vi "Bar Code Reader_v5.vi"() -> ()   [LabVIEW 2016]
uses:
  <vilib>/NXT/Block Support/NXT_OutputPort.ctl
  <vilib>/NXT/Block Support/NXT_InputPort.ctl
  <vilib>/NXT/Dual Mode Library/Sensors/EV3_Color_Color.vi
  <vilib>/NXT/NXTIO Xnodes/NXTIONodeSubVIs/NXTMoveMotors.vi
  <vilib>/NXT/NXTIO Xnodes/NXTIONodeSubVIs/NXTMotorRunDistance.vi
  <vilib>/NXT/Dual Mode Library/Waits/Wait_Num.vi
  <vilib>/NXT/Subs/LVHSConnector.ctl
  <vilib>/NXT/NXTIO Xnodes/AddressXNode/NXTIOAddress.xnode
  <vilib>/NXT/NXTIO Xnodes/NXTIOXNode/NXTIO.xnode
  <vilib>/NXT/LegoClasses/BrickReference/BrickReference.lvclass
panel:
  out "Error Message":string
  out "Total Marbles":dbl
  out "Small/HDPE 4":dbl
  out "Large/Steel 4":dbl
  out "Material 4":string
  out "Small/HDPE 3":dbl
  out "Large/Steel 3":dbl
  out "Material 3":string
  out "Small/HDPE 2":dbl
  out "Large/Steel 2":dbl
  out "Material 2":string
  out "Small/HDPE 1":dbl
  out "Large/Steel 1":dbl
  out "String 3":string
  out "String 2":string
  out "Material 1":string
  out "String":string
  out "Numeric":dbl
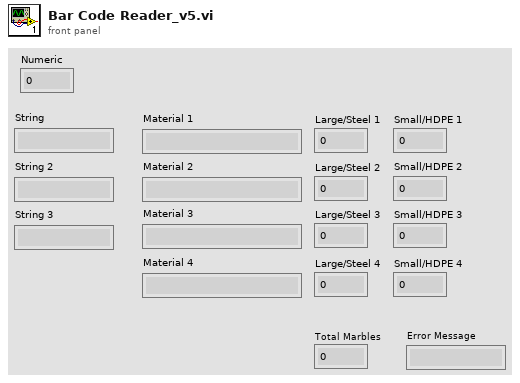
[diagram p1: front panel]
types:
  T1 = typedef "NXT_OutputPort.ctl" = u8
  T2 = typedef "ColorSensorColors.ctl" = enum16{"No Color", "Black", "Blue", "Green", "Yellow", "Red", "White", "Brown"}
  T3 = typedef "LVHSConnector.ctl" = refnum<class "BrickReference.lvclass">
  T4 = typedef "NXT_InputPort.ctl" = u32
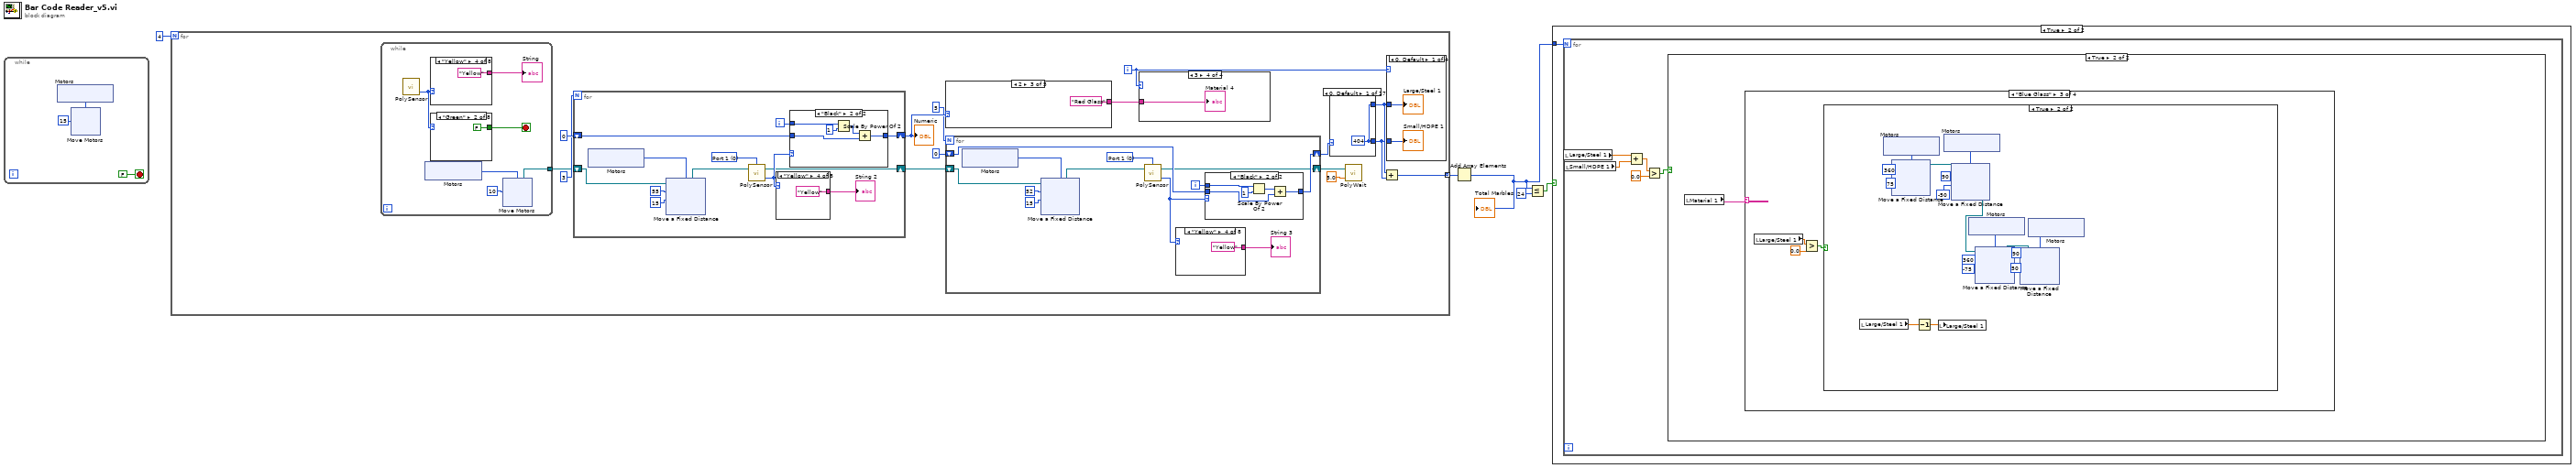
[diagram p0: block diagram]
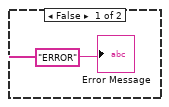
[diagram p2: hidden frame]
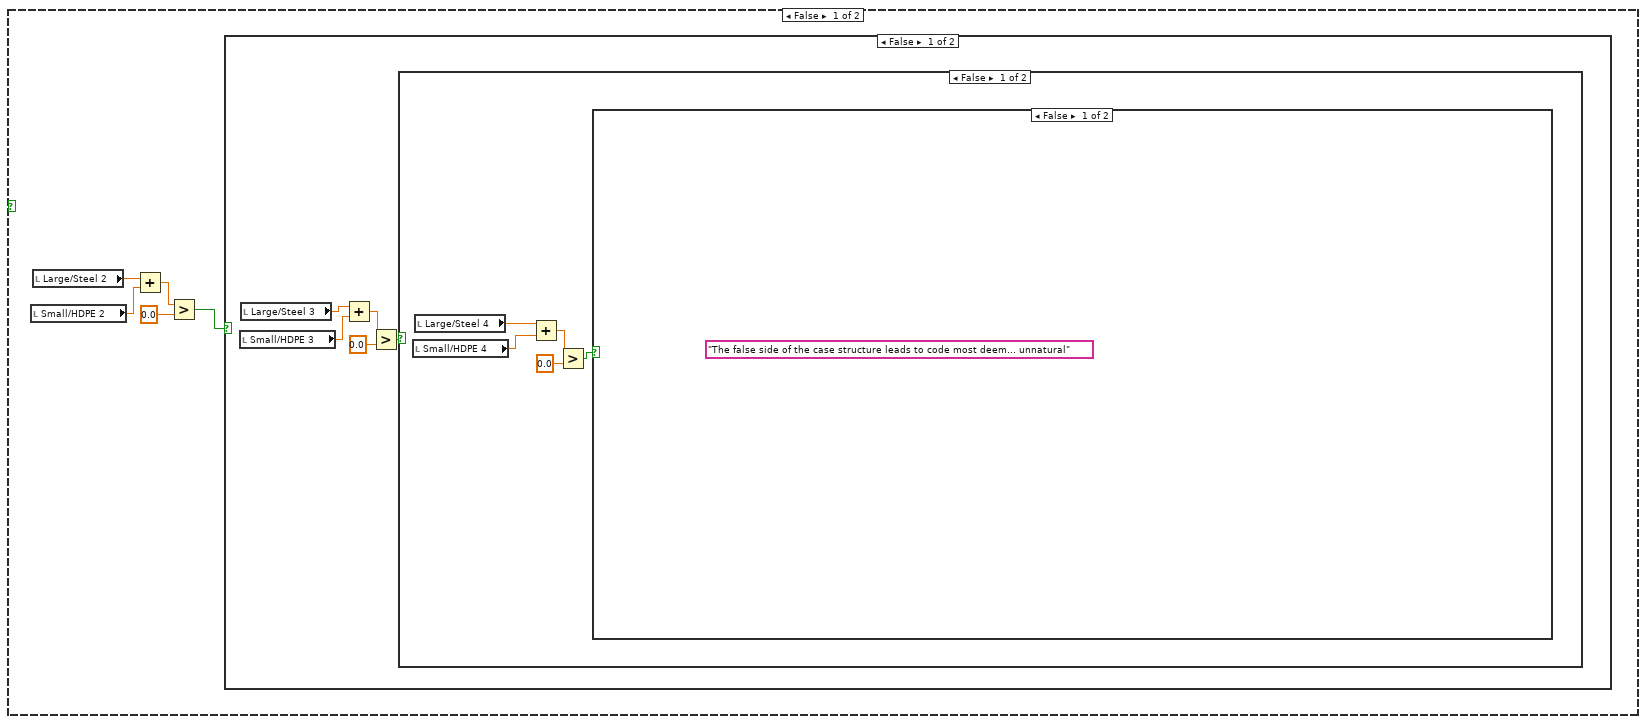
[diagram p3: hidden frame]
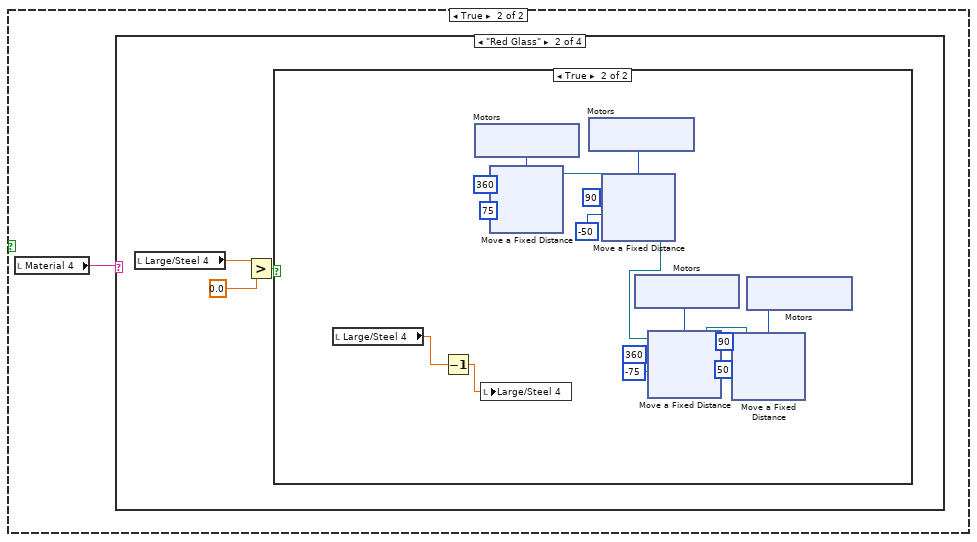
[diagram p4: hidden frame]
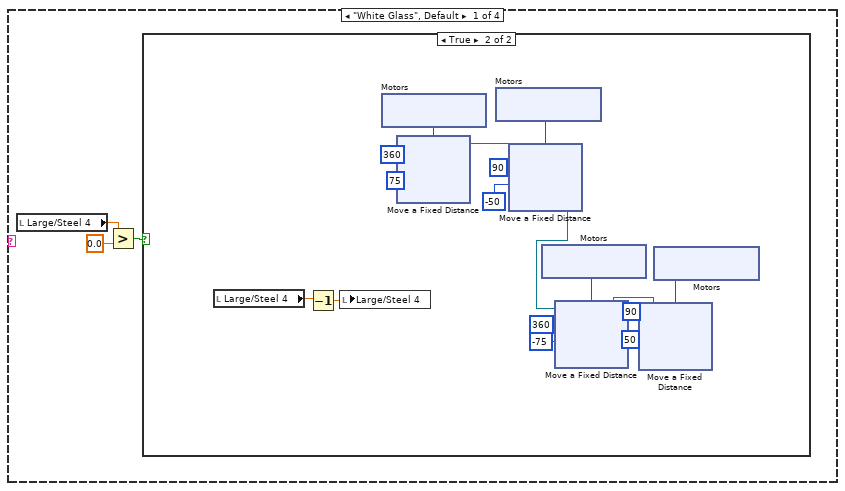
[diagram p5: hidden frame]
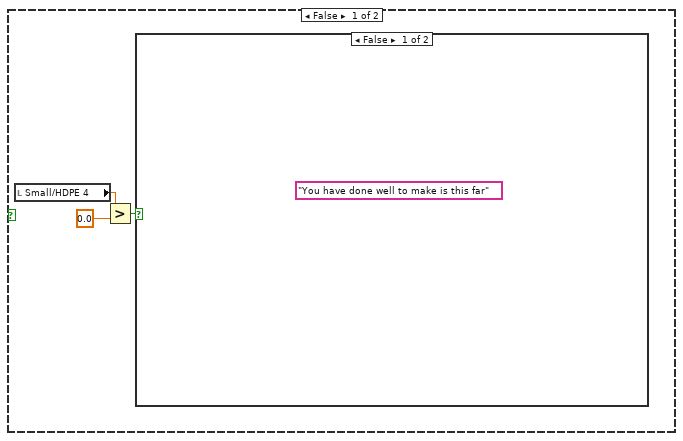
[diagram p6: hidden frame]
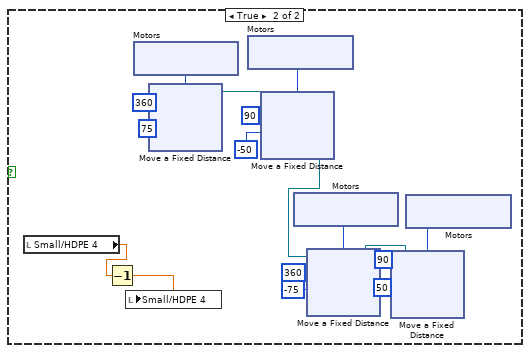
[diagram p7: hidden frame]
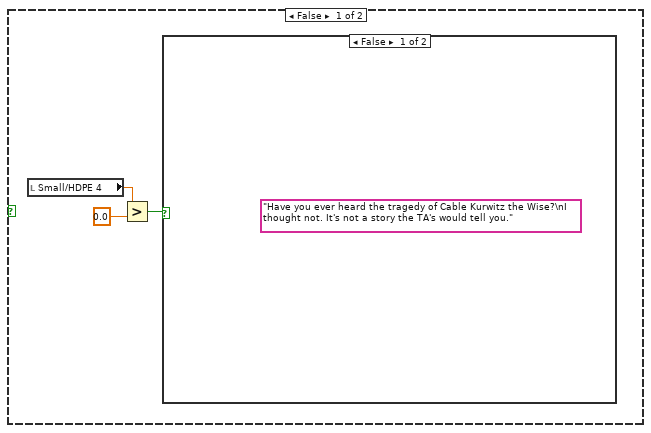
[diagram p8: hidden frame]
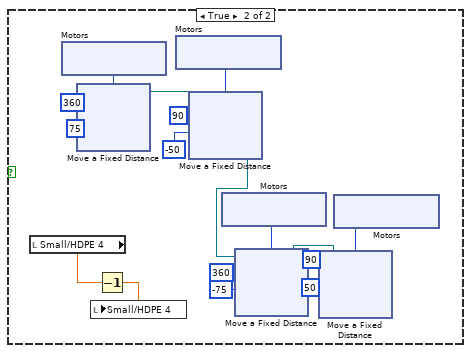
[diagram p9: hidden frame]
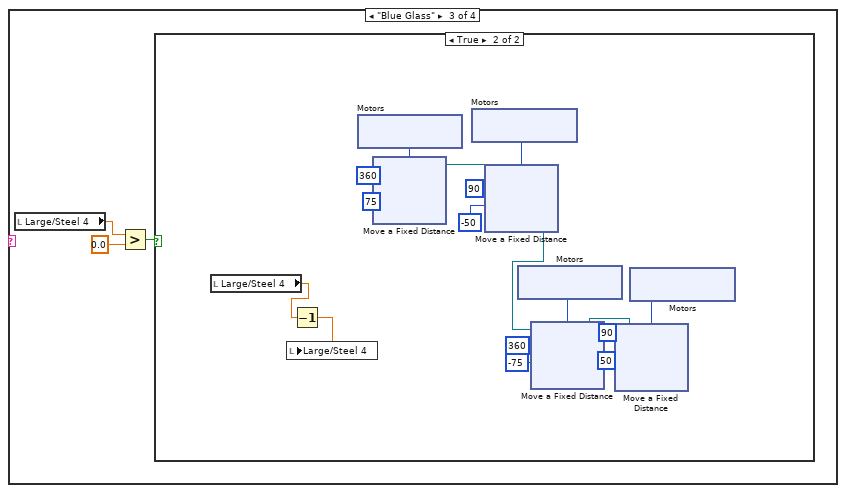
[diagram p10: hidden frame]
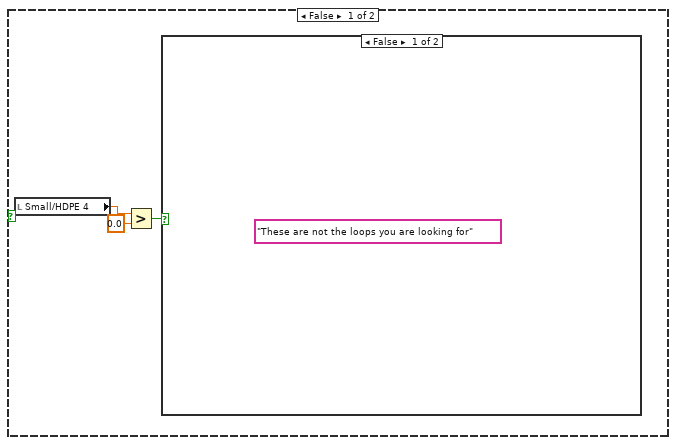
[diagram p11: hidden frame]
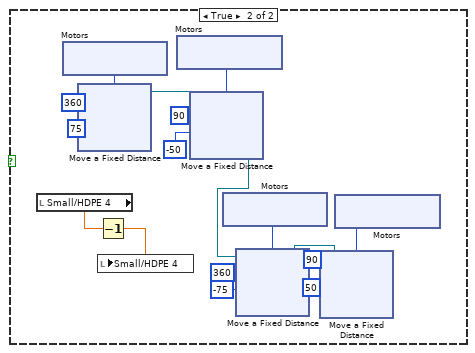
[diagram p12: hidden frame]
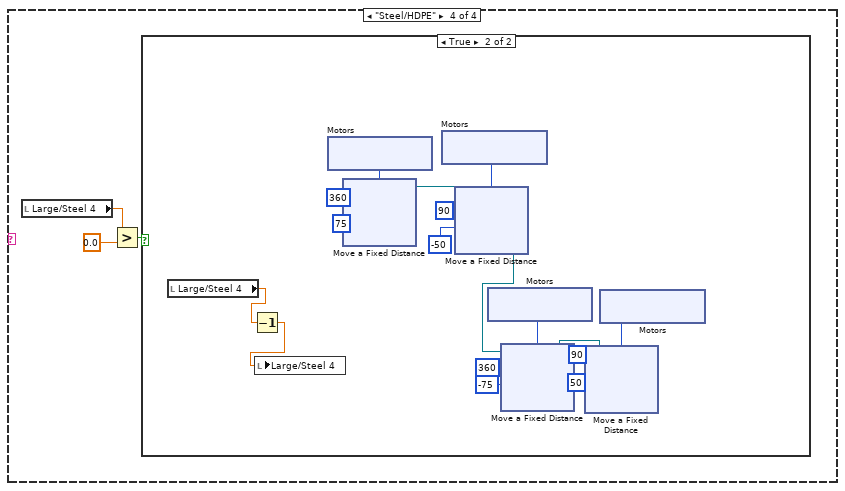
[diagram p13: hidden frame]
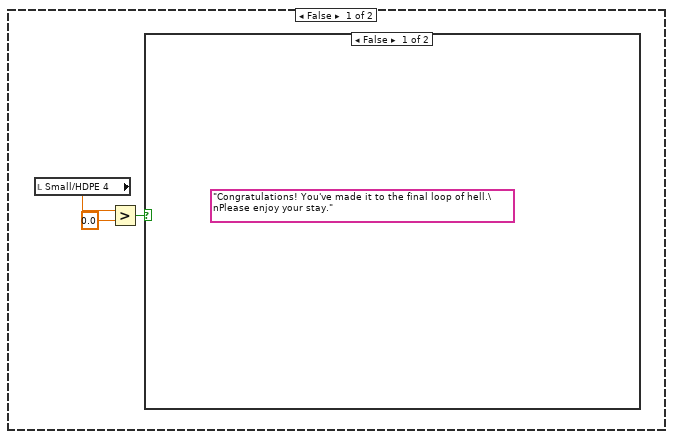
[diagram p14: hidden frame]
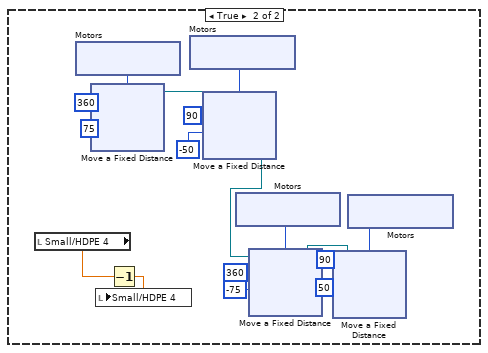
[diagram p15: hidden frame]
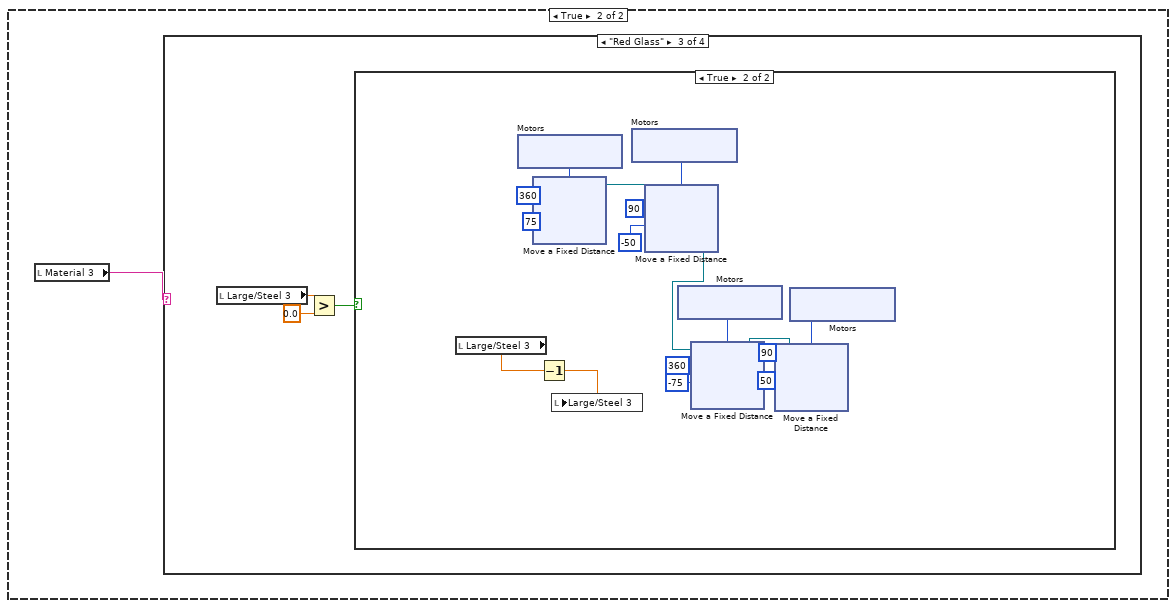
[diagram p16: hidden frame]
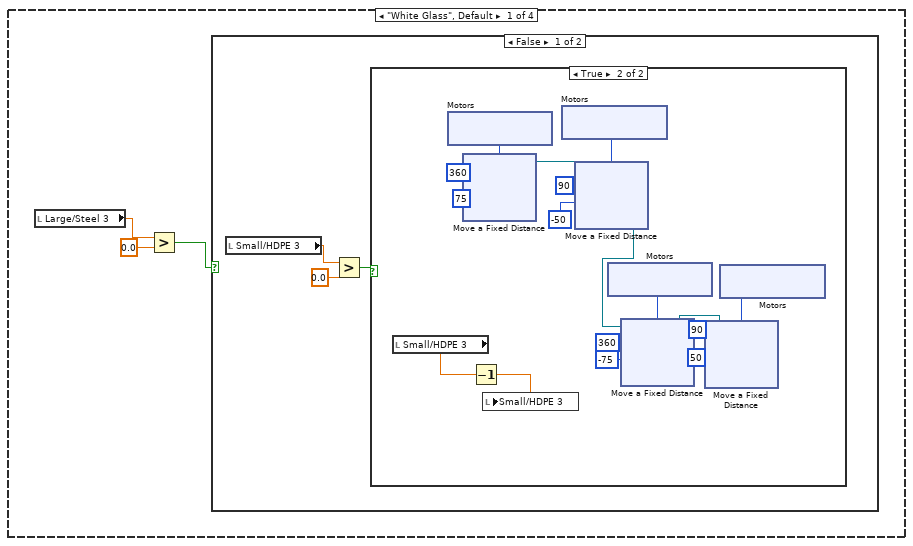
[diagram p17: hidden frame]
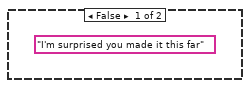
[diagram p18: hidden frame]
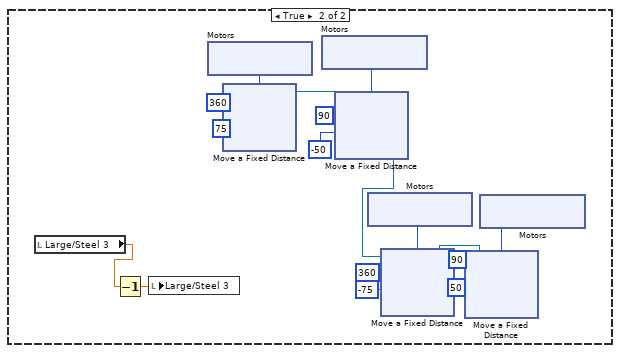
[diagram p19: hidden frame]
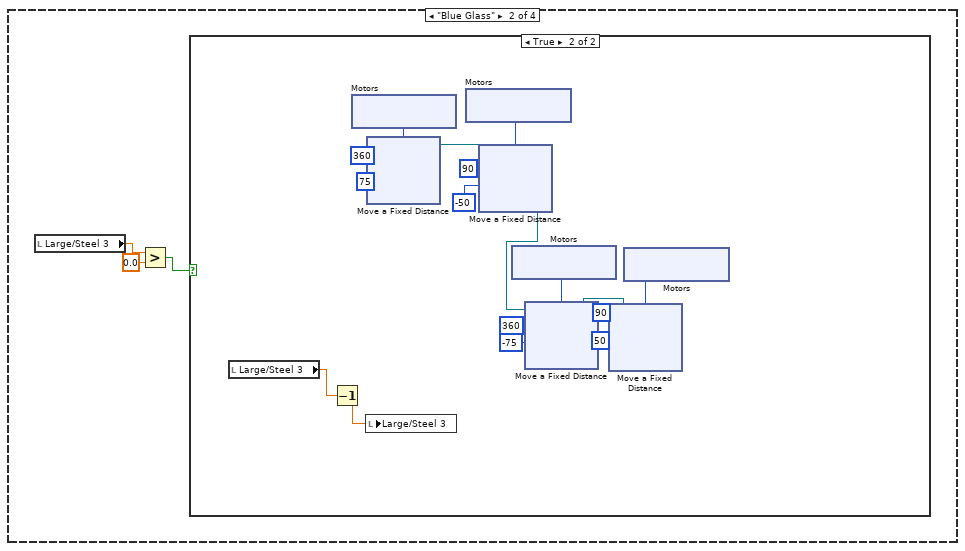
[diagram p20: hidden frame]
diagram:
  n1 = while {
    stop <- FALSE stop-if-true
    n2 = xnode "Motors"() -> ("Motor"=w6:T1)
    n3 = xnode "Move Motors"("Power/Speed 1"=i8 15, "Motors"=w6) -> ()  [unwired: 1 in, 1 out]
  }
  n4 = for {
    N: 4 -> [_]
    tunnel: [w17] -> w4 mode=indexing
    i -> [w22]
    n5 = while {
      tunnel: [w120] -> w29
      stop <- w124 stop-if-true
      n6 = call-poly <vilib>:"PolySensor.vi"() -> ("Detected Color"=w122:T2)  [unwired: 3 in, 1 out]
      n7 = xnode "Motors"() -> ("Motor"=w119:T1)
      n8 = case shown="\"Yellow\"" w122 {
        tunnel: ["No Color" "Blue" "Green" "Yellow" "Red" "White" "Brown" "Black"] -> w123
        frame "No Color", Default {
        }
        frame "Blue" {
        }
        frame "Green" {
        }
        frame "Yellow" {
        }
        frame "Red" {
        }
        frame "White" {
        }
        frame "Brown" {
        }
        frame "Black" {
        }
      }
      "String" <- w123
      n9 = case shown="\"Green\"" w122 {
        tunnel: [FALSE FALSE FALSE FALSE FALSE FALSE FALSE TRUE] -> w124
        frame "No Color", Default {
        }
        frame "Green" {
        }
        frame "Yellow" {
        }
        frame "Red" {
        }
        frame "White" {
        }
        frame "Brown" {
        }
        frame "Blue" {
        }
        frame "Black" {
        }
      }
      n10 = xnode "Move Motors"("Power/Speed 1"=i8 10, "Motors"=w119) -> ("NXT/EV3"=w120:T3)  [unwired: 1 in]
    }
    n11 = for {
      N: 3 -> [_]
      shift-right: [w160] -> w28
      shift-left: 0 -> [w159]
      shift-right: [w155] -> w24
      shift-left: w29 -> [w152]
      i -> [w156]
      w149 = T4 0 items=["Port 1", "Port 2", "Port 3", "Port 4"] ("Port (Port 1)")
      n12 = xnode "Motors"() -> ("Motor"=w150:T1)
      n13 = xnode "Move a Fixed Distance"("Speed 1"=i8 15, "Distance 1"=55, "Motors"=w150, "NXT/EV3"=w152) -> ("NXT/EV3"=w151:T3)
      n14 = call-poly <vilib>:"PolySensor.vi"("NXT/EV3"=w151, "Port (Port 1)"=w149) -> ("Detected Color"=w157:T2, "NXT/EV3"=w155:T3)  [unwired: 1 in]
      n15 = case shown="\"Yellow\"" w157 {
        tunnel: ["No Color" "Blue" "Green" "Yellow" "Red" "White" "Brown" "Black"] -> w158
        frame "No Color", Default {
        }
        frame "Blue" {
        }
        frame "Green" {
        }
        frame "Yellow" {
        }
        frame "Red" {
        }
        frame "White" {
        }
        frame "Brown" {
        }
        frame "Black" {
        }
      }
      "String 2" <- w158
      n16 = case shown="\"Black\"" w157 {
        tunnel: w156 -> [_ w184]
        tunnel: [w180 w182] -> w160
        tunnel: w159 -> [w180 w181]
        frame "White", Default {
        }
        frame "Black" {
          n17 = Scale By Power Of 2(n=w184, x=1) -> (x*2^n=w183:i32)
          n18 = Add(x=w183, y=w181) -> (x+y=w182:i32)
        }
      }
    }
    "Numeric" <- w28
    n19 = case shown="2" w28 {
      tunnel: ["Something has gone wrong" "White Glass" "Red Glass" "Blue Glass" "Steel/HDPE"] -> w27
      frame 0, Default {
      }
      frame 1 {
      }
      frame 2 {
      }
      frame 3 {
      }
      frame 4 {
      }
    }
    n20 = for {
      N: 5 -> [_]
      shift-right: [w88] -> w23
      shift-left: 0 -> [w87]
      shift-right: [w83] -> w21
      shift-left: w24 -> [w80]
      i -> [w84]
      w77 = T4 0 items=["Port 1", "Port 2", "Port 3", "Port 4"] ("Port (Port 1)")
      n21 = xnode "Motors"() -> ("Motor"=w78:T1)
      n22 = xnode "Move a Fixed Distance"("Speed 1"=i8 15, "Distance 1"=52, "Motors"=w78, "NXT/EV3"=w80) -> ("NXT/EV3"=w79:T3)
      n23 = call-poly <vilib>:"PolySensor.vi"("NXT/EV3"=w79, "Port (Port 1)"=w77) -> ("Detected Color"=w85:T2, "NXT/EV3"=w83:T3)  [unwired: 1 in]
      n24 = case shown="\"Yellow\"" w85 {
        tunnel: ["No Color" "Blue" "Green" "Yellow" "Red" "White" "Brown" "Black"] -> w86
        frame "No Color", Default {
        }
        frame "Blue" {
        }
        frame "Green" {
        }
        frame "Yellow" {
        }
        frame "Red" {
        }
        frame "White" {
        }
        frame "Brown" {
        }
        frame "Black" {
        }
      }
      "String 3" <- w86
      n25 = case shown="\"Black\"" w85 {
        tunnel: w84 -> [_ w112]
        tunnel: [w108 w110] -> w88
        tunnel: w87 -> [w108 w109]
        frame "White", Default {
        }
        frame "Black" {
          n26 = Scale By Power Of 2(n=w112, x=1) -> (x*2^n=w111:i32)
          n27 = Add(x=w111, y=w109) -> (x+y=w110:i32)
        }
      }
    }
    n28 = case shown="3" w22 {
      tunnel: w27 -> [w40 w41 w42 w43]
      frame 0, Default {
        "Material 1" <- w40
      }
      frame 1 {
        "Material 2" <- w41
      }
      frame 2 {
        "Material 3" <- w42
      }
      frame 3 {
        "Material 4" <- w43
      }
    }
    n29 = case shown="0, Default" w23 {
      tunnel: [w44 0 1 2 3 0 1 2 3 0 1 2 3 0 1 2 3] -> w19
      tunnel: [w44 0 0 0 0 1 1 1 1 2 2 2 2 3 3 3 3] -> w18
      frame 0, Default {
        w44 = 404
      }
      frame 1 {
      }
      frame 2 {
      }
      frame 3 {
      }
      frame 4 {
      }
      frame 5 {
      }
      frame 6 {
      }
      frame 7 {
      }
      frame 8 {
      }
      frame 9 {
      }
      frame 10 {
      }
      frame 11 {
      }
      frame 12 {
      }
      frame 13 {
      }
      frame 14 {
      }
      frame 15 {
      }
      frame 16 {
      }
    }
    n30 = call-poly <vilib>:"PolyWait.vi"("Time (1 sec)"=sgl 5.0, "NXT/EV3"=w21) -> ()  [unwired: 2 in, 1 out]
    n31 = Add(x=w19, y=w18) -> (x+y=w17:i32)
    n32 = case shown="0, Default" w22 {
      tunnel: w19 -> [w33 w34 w36 w38]
      tunnel: w18 -> [w32 w35 w37 w39]
      frame 0, Default {
        "Small/HDPE 1" <- w32
        "Large/Steel 1" <- w33
      }
      frame 1 {
        "Large/Steel 2" <- w34
        "Small/HDPE 2" <- w35
      }
      frame 2 {
        "Large/Steel 3" <- w36
        "Small/HDPE 3" <- w37
      }
      frame 3 {
        "Large/Steel 4" <- w38
        "Small/HDPE 4" <- w39
      }
    }
  }
  n33 = Add Array Elements(numeric array=w4) -> (sum=w3:i32)
  "Total Marbles" <- w3
  n34 = Less Or Equal?(x=w3, y=24) -> (x <= y?=w1:bool)
  n35 = case shown="True" w1 {
    tunnel: w3 -> [_ w187]
    frame False {
      "Error Message" <- "ERROR"
    }
    frame True {
      n36 = for {
        N: w187 -> [_]
        n37 = local read "Large/Steel 1"() -> (w192:dbl)
        n38 = local read "Small/HDPE 1"() -> (w191:dbl)
        n39 = Add(x=w192, y=w191) -> (x+y=w190:dbl)
        n40 = Greater?(x=w190, y=0.0) -> (0:w188:bool)
        n41 = case shown="True" w188 {
          frame False {
            n42 = local read "Small/HDPE 2"() -> (w195:dbl)
            n43 = local read "Large/Steel 2"() -> (w194:dbl)
            n44 = Add(x=w194, y=w195) -> (x+y=w197:dbl)
            n45 = Greater?(x=w197, y=0.0) -> (0:w193:bool)
            n46 = case shown="False" w193 {
              frame False {
                n47 = local read "Small/HDPE 3"() -> (w199:dbl)
                n48 = local read "Large/Steel 3"() -> (w200:dbl)
                n49 = Add(x=w200, y=w199) -> (x+y=w202:dbl)
                n50 = Greater?(x=w202, y=0.0) -> (0:w198:bool)
                n51 = case shown="False" w198 {
                  frame False {
                    n52 = local read "Small/HDPE 4"() -> (w204:dbl)
                    n53 = local read "Large/Steel 4"() -> (w205:dbl)
                    n54 = Add(x=w205, y=w204) -> (x+y=w207:dbl)
                    n55 = Greater?(x=w207, y=0.0) -> (0:w203:bool)
                    n56 = case shown="False" w203 {
                      frame False {
                        (unwired) "The false side of the case structure leads to code most deem... unnatural"
                      }
                      frame True {
                        n57 = local read "Material 4"() -> (w208:string)
                        n58 = case shown="\"Red Glass\"" w208 {
                          frame "White Glass", Default {
                            n59 = local read "Large/Steel 4"() -> (w210:dbl)
                            n60 = Greater?(x=w210, y=0.0) -> (0:w211:bool)
                            n61 = case shown="True" w211 {
                              frame False {
                                n62 = local read "Small/HDPE 4"() -> (w213:dbl)
                                n63 = Greater?(x=w213, y=0.0) -> (0:w214:bool)
                                n64 = case shown="False" w214 {
                                frame False {
                                (unwired) "You have done well to make is this far"
                                }
                                frame True {
                                n65 = local read "Small/HDPE 4"() -> (w231:dbl)
                                n66 = Decrement(x=w231) -> (x-1=w230:dbl)
                                n67 = local write "Small/HDPE 4"(w230) -> ()
                                n68 = xnode "Motors"() -> ("Motor"=w215:T1)
                                n69 = xnode "Move a Fixed Distance"("Speed 1"=i8 75, "Distance 1"=360, "Motors"=w215) -> ("NXT/EV3"=w218:T3)  [unwired: 1 in]
                                n70 = xnode "Motors"() -> ("Motor"=w219:T1)
                                n71 = xnode "Move a Fixed Distance"("Speed 1"=i8 -50, "Distance 1"=90, "Motors"=w219, "NXT/EV3"=w218) -> ("NXT/EV3"=w229:T3)
                                n72 = xnode "Motors"() -> ("Motor"=w225:T1)
                                n73 = xnode "Move a Fixed Distance"("Speed 1"=i8 -75, "Distance 1"=360, "Motors"=w225, "NXT/EV3"=w229) -> ("NXT/EV3"=w228:T3)
                                n74 = xnode "Motors"() -> ("Motor"=w222:T1)
                                n75 = xnode "Move a Fixed Distance"("Speed 1"=i8 50, "Distance 1"=90, "Motors"=w222, "NXT/EV3"=w228) -> ()  [unwired: 1 out]
                                }
                                }
                              }
                              frame True {
                                n76 = local read "Large/Steel 4"() -> (w292:dbl)
                                n77 = Decrement(x=w292) -> (x-1=w291:dbl)
                                n78 = local write "Large/Steel 4"(w291) -> ()
                                n79 = xnode "Motors"() -> ("Motor"=w276:T1)
                                n80 = xnode "Move a Fixed Distance"("Speed 1"=i8 75, "Distance 1"=360, "Motors"=w276) -> ("NXT/EV3"=w279:T3)  [unwired: 1 in]
                                n81 = xnode "Motors"() -> ("Motor"=w280:T1)
                                n82 = xnode "Move a Fixed Distance"("Speed 1"=i8 -50, "Distance 1"=90, "Motors"=w280, "NXT/EV3"=w279) -> ("NXT/EV3"=w290:T3)
                                n83 = xnode "Motors"() -> ("Motor"=w286:T1)
                                n84 = xnode "Move a Fixed Distance"("Speed 1"=i8 -75, "Distance 1"=360, "Motors"=w286, "NXT/EV3"=w290) -> ("NXT/EV3"=w289:T3)
                                n85 = xnode "Motors"() -> ("Motor"=w283:T1)
                                n86 = xnode "Move a Fixed Distance"("Speed 1"=i8 50, "Distance 1"=90, "Motors"=w283, "NXT/EV3"=w289) -> ()  [unwired: 1 out]
                              }
                            }
                          }
                          frame "Red Glass" {
                            n87 = local read "Large/Steel 4"() -> (w338:dbl)
                            n88 = Greater?(x=w338, y=0.0) -> (0:w339:bool)
                            n89 = case shown="True" w339 {
                              frame False {
                                n90 = local read "Small/HDPE 4"() -> (w340:dbl)
                                n91 = Greater?(x=w340, y=0.0) -> (0:w342:bool)
                                n92 = case shown="False" w342 {
                                frame False {
                                (unwired) "Have you ever heard the tragedy of Cable Kurwitz the Wise?\nI thought not. It's not a story the TA's would tell you."
                                }
                                frame True {
                                n93 = local read "Small/HDPE 4"() -> (w359:dbl)
                                n94 = xnode "Motors"() -> ("Motor"=w343:T1)
                                n95 = xnode "Move a Fixed Distance"("Speed 1"=i8 75, "Distance 1"=360, "Motors"=w343) -> ("NXT/EV3"=w346:T3)  [unwired: 1 in]
                                n96 = Decrement(x=w359) -> (x-1=w358:dbl)
                                n97 = local write "Small/HDPE 4"(w358) -> ()
                                n98 = xnode "Motors"() -> ("Motor"=w347:T1)
                                n99 = xnode "Move a Fixed Distance"("Speed 1"=i8 -50, "Distance 1"=90, "Motors"=w347, "NXT/EV3"=w346) -> ("NXT/EV3"=w357:T3)
                                n100 = xnode "Motors"() -> ("Motor"=w353:T1)
                                n101 = xnode "Move a Fixed Distance"("Speed 1"=i8 -75, "Distance 1"=360, "Motors"=w353, "NXT/EV3"=w357) -> ("NXT/EV3"=w356:T3)
                                n102 = xnode "Motors"() -> ("Motor"=w350:T1)
                                n103 = xnode "Move a Fixed Distance"("Speed 1"=i8 50, "Distance 1"=90, "Motors"=w350, "NXT/EV3"=w356) -> ()  [unwired: 1 out]
                                }
                                }
                              }
                              frame True {
                                n104 = local read "Large/Steel 4"() -> (w420:dbl)
                                n105 = Decrement(x=w420) -> (x-1=w419:dbl)
                                n106 = xnode "Motors"() -> ("Motor"=w404:T1)
                                n107 = local write "Large/Steel 4"(w419) -> ()
                                n108 = xnode "Move a Fixed Distance"("Speed 1"=i8 75, "Distance 1"=360, "Motors"=w404) -> ("NXT/EV3"=w407:T3)  [unwired: 1 in]
                                n109 = xnode "Motors"() -> ("Motor"=w408:T1)
                                n110 = xnode "Move a Fixed Distance"("Speed 1"=i8 -50, "Distance 1"=90, "Motors"=w408, "NXT/EV3"=w407) -> ("NXT/EV3"=w418:T3)
                                n111 = xnode "Motors"() -> ("Motor"=w414:T1)
                                n112 = xnode "Move a Fixed Distance"("Speed 1"=i8 -75, "Distance 1"=360, "Motors"=w414, "NXT/EV3"=w418) -> ("NXT/EV3"=w417:T3)
                                n113 = xnode "Motors"() -> ("Motor"=w411:T1)
                                n114 = xnode "Move a Fixed Distance"("Speed 1"=i8 50, "Distance 1"=90, "Motors"=w411, "NXT/EV3"=w417) -> ()  [unwired: 1 out]
                              }
                            }
                          }
                          frame "Blue Glass" {
                            n115 = local read "Large/Steel 4"() -> (w467:dbl)
                            n116 = Greater?(x=w467, y=0.0) -> (0:w466:bool)
                            n117 = case shown="True" w466 {
                              frame False {
                                n118 = local read "Small/HDPE 4"() -> (w469:dbl)
                                n119 = Greater?(x=w469, y=0.0) -> (0:w470:bool)
                                n120 = case shown="False" w470 {
                                frame False {
                                (unwired) "These are not the loops you are looking for"
                                }
                                frame True {
                                n121 = local read "Small/HDPE 4"() -> (w487:dbl)
                                n122 = xnode "Motors"() -> ("Motor"=w471:T1)
                                n123 = xnode "Move a Fixed Distance"("Speed 1"=i8 75, "Distance 1"=360, "Motors"=w471) -> ("NXT/EV3"=w474:T3)  [unwired: 1 in]
                                n124 = Decrement(x=w487) -> (x-1=w486:dbl)
                                n125 = local write "Small/HDPE 4"(w486) -> ()
                                n126 = xnode "Motors"() -> ("Motor"=w475:T1)
                                n127 = xnode "Move a Fixed Distance"("Speed 1"=i8 -50, "Distance 1"=90, "Motors"=w475, "NXT/EV3"=w474) -> ("NXT/EV3"=w485:T3)
                                n128 = xnode "Motors"() -> ("Motor"=w481:T1)
                                n129 = xnode "Move a Fixed Distance"("Speed 1"=i8 -75, "Distance 1"=360, "Motors"=w481, "NXT/EV3"=w485) -> ("NXT/EV3"=w484:T3)
                                n130 = xnode "Motors"() -> ("Motor"=w478:T1)
                                n131 = xnode "Move a Fixed Distance"("Speed 1"=i8 50, "Distance 1"=90, "Motors"=w478, "NXT/EV3"=w484) -> ()  [unwired: 1 out]
                                }
                                }
                              }
                              frame True {
                                n132 = local read "Large/Steel 4"() -> (w548:dbl)
                                n133 = Decrement(x=w548) -> (x-1=w547:dbl)
                                n134 = local write "Large/Steel 4"(w547) -> ()
                                n135 = xnode "Motors"() -> ("Motor"=w532:T1)
                                n136 = xnode "Move a Fixed Distance"("Speed 1"=i8 75, "Distance 1"=360, "Motors"=w532) -> ("NXT/EV3"=w535:T3)  [unwired: 1 in]
                                n137 = xnode "Motors"() -> ("Motor"=w536:T1)
                                n138 = xnode "Move a Fixed Distance"("Speed 1"=i8 -50, "Distance 1"=90, "Motors"=w536, "NXT/EV3"=w535) -> ("NXT/EV3"=w546:T3)
                                n139 = xnode "Motors"() -> ("Motor"=w542:T1)
                                n140 = xnode "Move a Fixed Distance"("Speed 1"=i8 -75, "Distance 1"=360, "Motors"=w542, "NXT/EV3"=w546) -> ("NXT/EV3"=w545:T3)
                                n141 = xnode "Motors"() -> ("Motor"=w539:T1)
                                n142 = xnode "Move a Fixed Distance"("Speed 1"=i8 50, "Distance 1"=90, "Motors"=w539, "NXT/EV3"=w545) -> ()  [unwired: 1 out]
                              }
                            }
                          }
                          frame "Steel/HDPE" {
                            n143 = local read "Large/Steel 4"() -> (w594:dbl)
                            n144 = Greater?(x=w594, y=0.0) -> (0:w595:bool)
                            n145 = case shown="True" w595 {
                              frame False {
                                n146 = local read "Small/HDPE 4"() -> (w597:dbl)
                                n147 = Greater?(x=w597, y=0.0) -> (0:w598:bool)
                                n148 = case shown="False" w598 {
                                frame False {
                                (unwired) "Congratulations! You've made it to the final loop of hell.\nPlease enjoy your stay."
                                }
                                frame True {
                                n149 = local read "Small/HDPE 4"() -> (w615:dbl)
                                n150 = xnode "Motors"() -> ("Motor"=w599:T1)
                                n151 = xnode "Move a Fixed Distance"("Speed 1"=i8 75, "Distance 1"=360, "Motors"=w599) -> ("NXT/EV3"=w602:T3)  [unwired: 1 in]
                                n152 = Decrement(x=w615) -> (x-1=w614:dbl)
                                n153 = local write "Small/HDPE 4"(w614) -> ()
                                n154 = xnode "Motors"() -> ("Motor"=w603:T1)
                                n155 = xnode "Move a Fixed Distance"("Speed 1"=i8 -50, "Distance 1"=90, "Motors"=w603, "NXT/EV3"=w602) -> ("NXT/EV3"=w613:T3)
                                n156 = xnode "Motors"() -> ("Motor"=w609:T1)
                                n157 = xnode "Move a Fixed Distance"("Speed 1"=i8 -75, "Distance 1"=360, "Motors"=w609, "NXT/EV3"=w613) -> ("NXT/EV3"=w612:T3)
                                n158 = xnode "Motors"() -> ("Motor"=w606:T1)
                                n159 = xnode "Move a Fixed Distance"("Speed 1"=i8 50, "Distance 1"=90, "Motors"=w606, "NXT/EV3"=w612) -> ()  [unwired: 1 out]
                                }
                                }
                              }
                              frame True {
                                n160 = local read "Large/Steel 4"() -> (w676:dbl)
                                n161 = Decrement(x=w676) -> (x-1=w675:dbl)
                                n162 = local write "Large/Steel 4"(w675) -> ()
                                n163 = xnode "Motors"() -> ("Motor"=w660:T1)
                                n164 = xnode "Move a Fixed Distance"("Speed 1"=i8 75, "Distance 1"=360, "Motors"=w660) -> ("NXT/EV3"=w663:T3)  [unwired: 1 in]
                                n165 = xnode "Motors"() -> ("Motor"=w664:T1)
                                n166 = xnode "Move a Fixed Distance"("Speed 1"=i8 -50, "Distance 1"=90, "Motors"=w664, "NXT/EV3"=w663) -> ("NXT/EV3"=w674:T3)
                                n167 = xnode "Motors"() -> ("Motor"=w670:T1)
                                n168 = xnode "Move a Fixed Distance"("Speed 1"=i8 -75, "Distance 1"=360, "Motors"=w670, "NXT/EV3"=w674) -> ("NXT/EV3"=w673:T3)
                                n169 = xnode "Motors"() -> ("Motor"=w667:T1)
                                n170 = xnode "Move a Fixed Distance"("Speed 1"=i8 50, "Distance 1"=90, "Motors"=w667, "NXT/EV3"=w673) -> ()  [unwired: 1 out]
                              }
                            }
                          }
                        }
                      }
                    }
                  }
                  frame True {
                    n171 = local read "Material 3"() -> (w721:string)
                    n172 = case shown="\"Red Glass\"" w721 {
                      frame "White Glass", Default {
                        n173 = local read "Large/Steel 3"() -> (w724:dbl)
                        n174 = Greater?(x=w724, y=0.0) -> (0:w722:bool)
                        n175 = case shown="False" w722 {
                          frame False {
                            n176 = local read "Small/HDPE 3"() -> (w726:dbl)
                            n177 = Greater?(x=w726, y=0.0) -> (0:w727:bool)
                            n178 = case shown="True" w727 {
                              frame False {
                                (unwired) "I'm surprised you made it this far"
                              }
                              frame True {
                                n179 = local read "Small/HDPE 3"() -> (w744:dbl)
                                n180 = xnode "Motors"() -> ("Motor"=w728:T1)
                                n181 = xnode "Move a Fixed Distance"("Speed 1"=i8 75, "Distance 1"=360, "Motors"=w728) -> ("NXT/EV3"=w731:T3)  [unwired: 1 in]
                                n182 = Decrement(x=w744) -> (x-1=w743:dbl)
                                n183 = local write "Small/HDPE 3"(w743) -> ()
                                n184 = xnode "Motors"() -> ("Motor"=w732:T1)
                                n185 = xnode "Move a Fixed Distance"("Speed 1"=i8 -50, "Distance 1"=90, "Motors"=w732, "NXT/EV3"=w731) -> ("NXT/EV3"=w742:T3)
                                n186 = xnode "Motors"() -> ("Motor"=w738:T1)
                                n187 = xnode "Move a Fixed Distance"("Speed 1"=i8 -75, "Distance 1"=360, "Motors"=w738, "NXT/EV3"=w742) -> ("NXT/EV3"=w741:T3)
                                n188 = xnode "Motors"() -> ("Motor"=w735:T1)
                                n189 = xnode "Move a Fixed Distance"("Speed 1"=i8 50, "Distance 1"=90, "Motors"=w735, "NXT/EV3"=w741) -> ()  [unwired: 1 out]
                              }
                            }
                          }
                          frame True {
                            n190 = local read "Large/Steel 3"() -> (w805:dbl)
                            n191 = Decrement(x=w805) -> (x-1=w804:dbl)
                            n192 = local write "Large/Steel 3"(w804) -> ()
                            n193 = xnode "Motors"() -> ("Motor"=w789:T1)
                            n194 = xnode "Move a Fixed Distance"("Speed 1"=i8 75, "Distance 1"=360, "Motors"=w789) -> ("NXT/EV3"=w792:T3)  [unwired: 1 in]
                            n195 = xnode "Motors"() -> ("Motor"=w793:T1)
                            n196 = xnode "Move a Fixed Distance"("Speed 1"=i8 -50, "Distance 1"=90, "Motors"=w793, "NXT/EV3"=w792) -> ("NXT/EV3"=w803:T3)
                            n197 = xnode "Motors"() -> ("Motor"=w799:T1)
                            n198 = xnode "Move a Fixed Distance"("Speed 1"=i8 -75, "Distance 1"=360, "Motors"=w799, "NXT/EV3"=w803) -> ("NXT/EV3"=w802:T3)
                            n199 = xnode "Motors"() -> ("Motor"=w796:T1)
                            n200 = xnode "Move a Fixed Distance"("Speed 1"=i8 50, "Distance 1"=90, "Motors"=w796, "NXT/EV3"=w802) -> ()  [unwired: 1 out]
                          }
                        }
                      }
                      frame "Blue Glass" {
                        n201 = local read "Large/Steel 3"() -> (w852:dbl)
                        n202 = Greater?(x=w852, y=0.0) -> (0:w850:bool)
                        n203 = case shown="True" w850 {
                          frame False {
                            n204 = local read "Small/HDPE 3"() -> (w855:dbl)
                            n205 = Greater?(x=w855, y=0.0) -> (0:w853:bool)
                            n206 = case shown="False" w853 {
                              frame False {
                                (unwired) "Welcome to the dark side of the case structure"
                              }
                              frame True {
                                n207 = local read "Small/HDPE 3"() -> (w872:dbl)
                                n208 = xnode "Motors"() -> ("Motor"=w856:T1)
                                n209 = Decrement(x=w872) -> (x-1=w871:dbl)
                                n210 = xnode "Move a Fixed Distance"("Speed 1"=i8 75, "Distance 1"=360, "Motors"=w856) -> ("NXT/EV3"=w859:T3)  [unwired: 1 in]
                                n211 = local write "Small/HDPE 3"(w871) -> ()
                                n212 = xnode "Motors"() -> ("Motor"=w860:T1)
                                n213 = xnode "Move a Fixed Distance"("Speed 1"=i8 -50, "Distance 1"=90, "Motors"=w860, "NXT/EV3"=w859) -> ("NXT/EV3"=w870:T3)
                                n214 = xnode "Motors"() -> ("Motor"=w866:T1)
                                n215 = xnode "Move a Fixed Distance"("Speed 1"=i8 -75, "Distance 1"=360, "Motors"=w866, "NXT/EV3"=w870) -> ("NXT/EV3"=w869:T3)
                                n216 = xnode "Motors"() -> ("Motor"=w863:T1)
                                n217 = xnode "Move a Fixed Distance"("Speed 1"=i8 50, "Distance 1"=90, "Motors"=w863, "NXT/EV3"=w869) -> ()  [unwired: 1 out]
                              }
                            }
                          }
                          frame True {
                            n218 = local read "Large/Steel 3"() -> (w933:dbl)
                            n219 = Decrement(x=w933) -> (x-1=w932:dbl)
                            n220 = xnode "Motors"() -> ("Motor"=w917:T1)
                            n221 = local write "Large/Steel 3"(w932) -> ()
                            n222 = xnode "Move a Fixed Distance"("Speed 1"=i8 75, "Distance 1"=360, "Motors"=w917) -> ("NXT/EV3"=w920:T3)  [unwired: 1 in]
                            n223 = xnode "Motors"() -> ("Motor"=w921:T1)
                            n224 = xnode "Move a Fixed Distance"("Speed 1"=i8 -50, "Distance 1"=90, "Motors"=w921, "NXT/EV3"=w920) -> ("NXT/EV3"=w931:T3)
                            n225 = xnode "Motors"() -> ("Motor"=w927:T1)
                            n226 = xnode "Move a Fixed Distance"("Speed 1"=i8 -75, "Distance 1"=360, "Motors"=w927, "NXT/EV3"=w931) -> ("NXT/EV3"=w930:T3)
                            n227 = xnode "Motors"() -> ("Motor"=w924:T1)
                            n228 = xnode "Move a Fixed Distance"("Speed 1"=i8 50, "Distance 1"=90, "Motors"=w924, "NXT/EV3"=w930) -> ()  [unwired: 1 out]
                          }
                        }
                      }
                      frame "Red Glass" {
                        n229 = local read "Large/Steel 3"() -> (w979:dbl)
                        n230 = Greater?(x=w979, y=0.0) -> (0:w980:bool)
                        n231 = case shown="True" w980 {
                          frame False {
                            n232 = local read "Small/HDPE 3"() -> (w982:dbl)
                            n233 = Greater?(x=w982, y=0.0) -> (0:w983:bool)
                            n234 = case shown="False" w983 {
                              frame False {
                                (unwired) "Two to the one to the one to the three"
                              }
                              frame True {
                                n235 = local read "Small/HDPE 3"() -> (w1000:dbl)
                                n236 = Decrement(x=w1000) -> (x-1=w999:dbl)
                                n237 = local write "Small/HDPE 3"(w999) -> ()
                                n238 = xnode "Motors"() -> ("Motor"=w984:T1)
                                n239 = xnode "Move a Fixed Distance"("Speed 1"=i8 75, "Distance 1"=360, "Motors"=w984) -> ("NXT/EV3"=w987:T3)  [unwired: 1 in]
                                n240 = xnode "Motors"() -> ("Motor"=w988:T1)
                                n241 = xnode "Move a Fixed Distance"("Speed 1"=i8 -50, "Distance 1"=90, "Motors"=w988, "NXT/EV3"=w987) -> ("NXT/EV3"=w998:T3)
                                n242 = xnode "Motors"() -> ("Motor"=w994:T1)
                                n243 = xnode "Move a Fixed Distance"("Speed 1"=i8 -75, "Distance 1"=360, "Motors"=w994, "NXT/EV3"=w998) -> ("NXT/EV3"=w997:T3)
                                n244 = xnode "Motors"() -> ("Motor"=w991:T1)
                                n245 = xnode "Move a Fixed Distance"("Speed 1"=i8 50, "Distance 1"=90, "Motors"=w991, "NXT/EV3"=w997) -> ()  [unwired: 1 out]
                              }
                            }
                          }
                          frame True {
                            n246 = local read "Large/Steel 3"() -> (w1061:dbl)
                            n247 = xnode "Motors"() -> ("Motor"=w1045:T1)
                            n248 = xnode "Move a Fixed Distance"("Speed 1"=i8 75, "Distance 1"=360, "Motors"=w1045) -> ("NXT/EV3"=w1048:T3)  [unwired: 1 in]
                            n249 = Decrement(x=w1061) -> (x-1=w1060:dbl)
                            n250 = local write "Large/Steel 3"(w1060) -> ()
                            n251 = xnode "Motors"() -> ("Motor"=w1049:T1)
                            n252 = xnode "Move a Fixed Distance"("Speed 1"=i8 -50, "Distance 1"=90, "Motors"=w1049, "NXT/EV3"=w1048) -> ("NXT/EV3"=w1059:T3)
                            n253 = xnode "Motors"() -> ("Motor"=w1055:T1)
                            n254 = xnode "Move a Fixed Distance"("Speed 1"=i8 -75, "Distance 1"=360, "Motors"=w1055, "NXT/EV3"=w1059) -> ("NXT/EV3"=w1058:T3)
                            n255 = xnode "Motors"() -> ("Motor"=w1052:T1)
                            n256 = xnode "Move a Fixed Distance"("Speed 1"=i8 50, "Distance 1"=90, "Motors"=w1052, "NXT/EV3"=w1058) -> ()  [unwired: 1 out]
                          }
                        }
                      }
                      frame "Steel/HDPE" {
                        n257 = local read "Large/Steel 3"() -> (w1107:dbl)
                        n258 = Greater?(x=w1107, y=0.0) -> (0:w1108:bool)
                        n259 = case shown="True" w1108 {
                          frame False {
                            n260 = local read "Small/HDPE 3"() -> (w1110:dbl)
                            n261 = Greater?(x=w1110, y=0.0) -> (0:w1111:bool)
                            n262 = case shown="True" w1111 {
                              frame False {
                                (unwired) "labview wouldnt let me copy the variables successfully\nso I had to write every single case structure by hand."
                              }
                              frame True {
                                n263 = local read "Small/HDPE 3"() -> (w1128:dbl)
                                n264 = xnode "Motors"() -> ("Motor"=w1112:T1)
                                n265 = Decrement(x=w1128) -> (x-1=w1127:dbl)
                                n266 = xnode "Move a Fixed Distance"("Speed 1"=i8 75, "Distance 1"=360, "Motors"=w1112) -> ("NXT/EV3"=w1115:T3)  [unwired: 1 in]
                                n267 = local write "Small/HDPE 3"(w1127) -> ()
                                n268 = xnode "Motors"() -> ("Motor"=w1116:T1)
                                n269 = xnode "Move a Fixed Distance"("Speed 1"=i8 -50, "Distance 1"=90, "Motors"=w1116, "NXT/EV3"=w1115) -> ("NXT/EV3"=w1126:T3)
                                n270 = xnode "Motors"() -> ("Motor"=w1122:T1)
                                n271 = xnode "Move a Fixed Distance"("Speed 1"=i8 -75, "Distance 1"=360, "Motors"=w1122, "NXT/EV3"=w1126) -> ("NXT/EV3"=w1125:T3)
                                n272 = xnode "Motors"() -> ("Motor"=w1119:T1)
                                n273 = xnode "Move a Fixed Distance"("Speed 1"=i8 50, "Distance 1"=90, "Motors"=w1119, "NXT/EV3"=w1125) -> ()  [unwired: 1 out]
                              }
                            }
                          }
                          frame True {
                            n274 = local read "Large/Steel 3"() -> (w1189:dbl)
                            n275 = Decrement(x=w1189) -> (x-1=w1188:dbl)
                            n276 = xnode "Motors"() -> ("Motor"=w1173:T1)
                            n277 = xnode "Move a Fixed Distance"("Speed 1"=i8 75, "Distance 1"=360, "Motors"=w1173) -> ("NXT/EV3"=w1176:T3)  [unwired: 1 in]
                            n278 = local write "Large/Steel 3"(w1188) -> ()
                            n279 = xnode "Motors"() -> ("Motor"=w1177:T1)
                            n280 = xnode "Move a Fixed Distance"("Speed 1"=i8 -50, "Distance 1"=90, "Motors"=w1177, "NXT/EV3"=w1176) -> ("NXT/EV3"=w1187:T3)
                            n281 = xnode "Motors"() -> ("Motor"=w1183:T1)
                            n282 = xnode "Move a Fixed Distance"("Speed 1"=i8 -75, "Distance 1"=360, "Motors"=w1183, "NXT/EV3"=w1187) -> ("NXT/EV3"=w1186:T3)
                            n283 = xnode "Motors"() -> ("Motor"=w1180:T1)
                            n284 = xnode "Move a Fixed Distance"("Speed 1"=i8 50, "Distance 1"=90, "Motors"=w1180, "NXT/EV3"=w1186) -> ()  [unwired: 1 out]
                          }
                        }
                      }
                    }
                  }
                }
              }
              frame True {
                n285 = local read "Material 2"() -> (w1234:string)
                n286 = case shown="\"Steel/HDPE\"" w1234 {
                  frame "White Glass", Default {
                    n287 = local read "Large/Steel 2"() -> (w1237:dbl)
                    n288 = Greater?(x=w1237, y=0.0) -> (0:w1235:bool)
                    n289 = case shown="False" w1235 {
                      frame False {
                        n290 = local read "Small/HDPE 2"() -> (w1240:dbl)
                        n291 = Greater?(x=w1240, y=0.0) -> (0:w1238:bool)
                        n292 = case shown="True" w1238 {
                          frame False {
                            (unwired) "howdy random TA"
                          }
                          frame True {
                            n293 = local read "Small/HDPE 2"() -> (w1257:dbl)
                            n294 = Decrement(x=w1257) -> (x-1=w1256:dbl)
                            n295 = local write "Small/HDPE 2"(w1256) -> ()
                            n296 = xnode "Motors"() -> ("Motor"=w1241:T1)
                            n297 = xnode "Move a Fixed Distance"("Speed 1"=i8 75, "Distance 1"=360, "Motors"=w1241) -> ("NXT/EV3"=w1244:T3)  [unwired: 1 in]
                            n298 = xnode "Motors"() -> ("Motor"=w1245:T1)
                            n299 = xnode "Move a Fixed Distance"("Speed 1"=i8 -50, "Distance 1"=90, "Motors"=w1245, "NXT/EV3"=w1244) -> ("NXT/EV3"=w1255:T3)
                            n300 = xnode "Motors"() -> ("Motor"=w1251:T1)
                            n301 = xnode "Move a Fixed Distance"("Speed 1"=i8 -75, "Distance 1"=360, "Motors"=w1251, "NXT/EV3"=w1255) -> ("NXT/EV3"=w1254:T3)
                            n302 = xnode "Motors"() -> ("Motor"=w1248:T1)
                            n303 = xnode "Move a Fixed Distance"("Speed 1"=i8 50, "Distance 1"=90, "Motors"=w1248, "NXT/EV3"=w1254) -> ()  [unwired: 1 out]
                          }
                        }
                      }
                      frame True {
                        n304 = local read "Large/Steel 2"() -> (w1318:dbl)
                        n305 = Decrement(x=w1318) -> (x-1=w1317:dbl)
                        n306 = local write "Large/Steel 2"(w1317) -> ()
                        n307 = xnode "Motors"() -> ("Motor"=w1302:T1)
                        n308 = xnode "Move a Fixed Distance"("Speed 1"=i8 75, "Distance 1"=360, "Motors"=w1302) -> ("NXT/EV3"=w1305:T3)  [unwired: 1 in]
                        n309 = xnode "Motors"() -> ("Motor"=w1306:T1)
                        n310 = xnode "Move a Fixed Distance"("Speed 1"=i8 -50, "Distance 1"=90, "Motors"=w1306, "NXT/EV3"=w1305) -> ("NXT/EV3"=w1316:T3)
                        n311 = xnode "Motors"() -> ("Motor"=w1312:T1)
                        n312 = xnode "Move a Fixed Distance"("Speed 1"=i8 -75, "Distance 1"=360, "Motors"=w1312, "NXT/EV3"=w1316) -> ("NXT/EV3"=w1315:T3)
                        n313 = xnode "Motors"() -> ("Motor"=w1309:T1)
                        n314 = xnode "Move a Fixed Distance"("Speed 1"=i8 50, "Distance 1"=90, "Motors"=w1309, "NXT/EV3"=w1315) -> ()  [unwired: 1 out]
                      }
                    }
                  }
                  frame "Blue Glass" {
                    n315 = local read "Large/Steel 2"() -> (w1365:dbl)
                    n316 = Greater?(x=w1365, y=0.0) -> (0:w1364:bool)
                    n317 = case shown="True" w1364 {
                      frame True {
                        n318 = local read "Large/Steel 2"() -> (w1382:dbl)
                        n319 = Decrement(x=w1382) -> (x-1=w1381:dbl)
                        n320 = local write "Large/Steel 2"(w1381) -> ()
                        n321 = xnode "Motors"() -> ("Motor"=w1366:T1)
                        n322 = xnode "Move a Fixed Distance"("Speed 1"=i8 75, "Distance 1"=360, "Motors"=w1366) -> ("NXT/EV3"=w1369:T3)  [unwired: 1 in]
                        n323 = xnode "Motors"() -> ("Motor"=w1370:T1)
                        n324 = xnode "Move a Fixed Distance"("Speed 1"=i8 -50, "Distance 1"=90, "Motors"=w1370, "NXT/EV3"=w1369) -> ("NXT/EV3"=w1380:T3)
                        n325 = xnode "Motors"() -> ("Motor"=w1376:T1)
                        n326 = xnode "Move a Fixed Distance"("Speed 1"=i8 -75, "Distance 1"=360, "Motors"=w1376, "NXT/EV3"=w1380) -> ("NXT/EV3"=w1379:T3)
                        n327 = xnode "Motors"() -> ("Motor"=w1373:T1)
                        n328 = xnode "Move a Fixed Distance"("Speed 1"=i8 50, "Distance 1"=90, "Motors"=w1373, "NXT/EV3"=w1379) -> ()  [unwired: 1 out]
                      }
                      frame False {
                        n329 = local read "Small/HDPE 2"() -> (w1429:dbl)
                        n330 = Greater?(x=w1429, y=0.0) -> (0:w1427:bool)
                        n331 = case shown="True" w1427 {
                          frame False {
                            (unwired) "This statement is false"
                          }
                          frame True {
                            n332 = local read "Small/HDPE 2"() -> (w1446:dbl)
                            n333 = Decrement(x=w1446) -> (x-1=w1445:dbl)
                            n334 = local write "Small/HDPE 2"(w1445) -> ()
                            n335 = xnode "Motors"() -> ("Motor"=w1430:T1)
                            n336 = xnode "Move a Fixed Distance"("Speed 1"=i8 75, "Distance 1"=360, "Motors"=w1430) -> ("NXT/EV3"=w1433:T3)  [unwired: 1 in]
                            n337 = xnode "Motors"() -> ("Motor"=w1434:T1)
                            n338 = xnode "Move a Fixed Distance"("Speed 1"=i8 -50, "Distance 1"=90, "Motors"=w1434, "NXT/EV3"=w1433) -> ("NXT/EV3"=w1444:T3)
                            n339 = xnode "Motors"() -> ("Motor"=w1440:T1)
                            n340 = xnode "Move a Fixed Distance"("Speed 1"=i8 -75, "Distance 1"=360, "Motors"=w1440, "NXT/EV3"=w1444) -> ("NXT/EV3"=w1443:T3)
                            n341 = xnode "Motors"() -> ("Motor"=w1437:T1)
                            n342 = xnode "Move a Fixed Distance"("Speed 1"=i8 50, "Distance 1"=90, "Motors"=w1437, "NXT/EV3"=w1443) -> ()  [unwired: 1 out]
                          }
                        }
                      }
                    }
                  }
                  frame "Red Glass" {
                    n343 = local read "Large/Steel 2"() -> (w1493:dbl)
                    n344 = Greater?(x=w1493, y=0.0) -> (0:w1491:bool)
                    n345 = case shown="False" w1491 {
                      frame False {
                        n346 = local read "Small/HDPE 2"() -> (w1496:dbl)
                        n347 = Greater?(x=w1496, y=0.0) -> (0:w1494:bool)
                        n348 = case shown="True" w1494 {
                          frame False {
                            (unwired) "I hate everything\n"
                          }
                          frame True {
                            n349 = local read "Small/HDPE 2"() -> (w1513:dbl)
                            n350 = xnode "Motors"() -> ("Motor"=w1497:T1)
                            n351 = xnode "Move a Fixed Distance"("Speed 1"=i8 75, "Distance 1"=360, "Motors"=w1497) -> ("NXT/EV3"=w1500:T3)  [unwired: 1 in]
                            n352 = Decrement(x=w1513) -> (x-1=w1512:dbl)
                            n353 = local write "Small/HDPE 2"(w1512) -> ()
                            n354 = xnode "Motors"() -> ("Motor"=w1501:T1)
                            n355 = xnode "Move a Fixed Distance"("Speed 1"=i8 -50, "Distance 1"=90, "Motors"=w1501, "NXT/EV3"=w1500) -> ("NXT/EV3"=w1511:T3)
                            n356 = xnode "Motors"() -> ("Motor"=w1507:T1)
                            n357 = xnode "Move a Fixed Distance"("Speed 1"=i8 -75, "Distance 1"=360, "Motors"=w1507, "NXT/EV3"=w1511) -> ("NXT/EV3"=w1510:T3)
                            n358 = xnode "Motors"() -> ("Motor"=w1504:T1)
                            n359 = xnode "Move a Fixed Distance"("Speed 1"=i8 50, "Distance 1"=90, "Motors"=w1504, "NXT/EV3"=w1510) -> ()  [unwired: 1 out]
                          }
                        }
                      }
                      frame True {
                        n360 = local read "Large/Steel 2"() -> (w1574:dbl)
                        n361 = Decrement(x=w1574) -> (x-1=w1573:dbl)
                        n362 = local write "Large/Steel 2"(w1573) -> ()
                        n363 = xnode "Motors"() -> ("Motor"=w1558:T1)
                        n364 = xnode "Move a Fixed Distance"("Speed 1"=i8 75, "Distance 1"=360, "Motors"=w1558) -> ("NXT/EV3"=w1561:T3)  [unwired: 1 in]
                        n365 = xnode "Motors"() -> ("Motor"=w1562:T1)
                        n366 = xnode "Move a Fixed Distance"("Speed 1"=i8 -50, "Distance 1"=90, "Motors"=w1562, "NXT/EV3"=w1561) -> ("NXT/EV3"=w1572:T3)
                        n367 = xnode "Motors"() -> ("Motor"=w1568:T1)
                        n368 = xnode "Move a Fixed Distance"("Speed 1"=i8 -75, "Distance 1"=360, "Motors"=w1568, "NXT/EV3"=w1572) -> ("NXT/EV3"=w1571:T3)
                        n369 = xnode "Motors"() -> ("Motor"=w1565:T1)
                        n370 = xnode "Move a Fixed Distance"("Speed 1"=i8 50, "Distance 1"=90, "Motors"=w1565, "NXT/EV3"=w1571) -> ()  [unwired: 1 out]
                      }
                    }
                  }
                  frame "Steel/HDPE" {
                    n371 = local read "Large/Steel 2"() -> (w1621:dbl)
                    n372 = Greater?(x=w1621, y=0.0) -> (0:w1619:bool)
                    n373 = case shown="True" w1619 {
                      frame False {
                        n374 = local read "Small/HDPE 2"() -> (w1624:dbl)
                        n375 = Greater?(x=w1624, y=0.0) -> (0:w1622:bool)
                        n376 = case shown="True" w1622 {
                          frame False {
                            (unwired) "I've lost all my marbles"
                          }
                          frame True {
                            n377 = local read "Small/HDPE 2"() -> (w1641:dbl)
                            n378 = xnode "Motors"() -> ("Motor"=w1625:T1)
                            n379 = xnode "Move a Fixed Distance"("Speed 1"=i8 75, "Distance 1"=360, "Motors"=w1625) -> ("NXT/EV3"=w1628:T3)  [unwired: 1 in]
                            n380 = Decrement(x=w1641) -> (x-1=w1640:dbl)
                            n381 = local write "Small/HDPE 2"(w1640) -> ()
                            n382 = xnode "Motors"() -> ("Motor"=w1629:T1)
                            n383 = xnode "Move a Fixed Distance"("Speed 1"=i8 -50, "Distance 1"=90, "Motors"=w1629, "NXT/EV3"=w1628) -> ("NXT/EV3"=w1639:T3)
                            n384 = xnode "Motors"() -> ("Motor"=w1635:T1)
                            n385 = xnode "Move a Fixed Distance"("Speed 1"=i8 -75, "Distance 1"=360, "Motors"=w1635, "NXT/EV3"=w1639) -> ("NXT/EV3"=w1638:T3)
                            n386 = xnode "Motors"() -> ("Motor"=w1632:T1)
                            n387 = xnode "Move a Fixed Distance"("Speed 1"=i8 50, "Distance 1"=90, "Motors"=w1632, "NXT/EV3"=w1638) -> ()  [unwired: 1 out]
                          }
                        }
                      }
                      frame True {
                        n388 = local read "Large/Steel 2"() -> (w1702:dbl)
                        n389 = Decrement(x=w1702) -> (x-1=w1701:dbl)
                        n390 = local write "Large/Steel 2"(w1701) -> ()
                        n391 = xnode "Motors"() -> ("Motor"=w1686:T1)
                        n392 = xnode "Move a Fixed Distance"("Speed 1"=i8 75, "Distance 1"=360, "Motors"=w1686) -> ("NXT/EV3"=w1689:T3)  [unwired: 1 in]
                        n393 = xnode "Motors"() -> ("Motor"=w1690:T1)
                        n394 = xnode "Move a Fixed Distance"("Speed 1"=i8 -50, "Distance 1"=90, "Motors"=w1690, "NXT/EV3"=w1689) -> ("NXT/EV3"=w1700:T3)
                        n395 = xnode "Motors"() -> ("Motor"=w1696:T1)
                        n396 = xnode "Move a Fixed Distance"("Speed 1"=i8 -75, "Distance 1"=360, "Motors"=w1696, "NXT/EV3"=w1700) -> ("NXT/EV3"=w1699:T3)
                        n397 = xnode "Motors"() -> ("Motor"=w1693:T1)
                        n398 = xnode "Move a Fixed Distance"("Speed 1"=i8 50, "Distance 1"=90, "Motors"=w1693, "NXT/EV3"=w1699) -> ()  [unwired: 1 out]
                      }
                    }
                  }
                }
              }
            }
          }
          frame True {
            n399 = local read "Material 1"() -> (w1747:string)
            n400 = case shown="\"Blue Glass\"" w1747 {
              frame "White Glass", Default {
                n401 = local read "Large/Steel 1"() -> (w1749:dbl)
                n402 = Greater?(x=w1749, y=0.0) -> (0:w1748:bool)
                n403 = case shown="False" w1748 {
                  frame False {
                    n404 = local read "Small/HDPE 1"() -> (w1752:dbl)
                    n405 = Greater?(x=w1752, y=0.0) -> (0:w1751:bool)
                    n406 = case shown="True" w1751 {
                      frame False {
                        (unwired) "go away"
                      }
                      frame True {
                        n407 = local read "Small/HDPE 1"() -> (w1770:dbl)
                        n408 = xnode "Motors"() -> ("Motor"=w1754:T1)
                        n409 = xnode "Move a Fixed Distance"("Speed 1"=i8 75, "Distance 1"=360, "Motors"=w1754) -> ("NXT/EV3"=w1757:T3)  [unwired: 1 in]
                        n410 = Decrement(x=w1770) -> (x-1=w1769:dbl)
                        n411 = local write "Small/HDPE 1"(w1769) -> ()
                        n412 = xnode "Motors"() -> ("Motor"=w1758:T1)
                        n413 = xnode "Move a Fixed Distance"("Speed 1"=i8 -50, "Distance 1"=90, "Motors"=w1758, "NXT/EV3"=w1757) -> ("NXT/EV3"=w1768:T3)
                        n414 = xnode "Motors"() -> ("Motor"=w1764:T1)
                        n415 = xnode "Move a Fixed Distance"("Speed 1"=i8 -75, "Distance 1"=360, "Motors"=w1764, "NXT/EV3"=w1768) -> ("NXT/EV3"=w1767:T3)
                        n416 = xnode "Motors"() -> ("Motor"=w1761:T1)
                        n417 = xnode "Move a Fixed Distance"("Speed 1"=i8 50, "Distance 1"=90, "Motors"=w1761, "NXT/EV3"=w1767) -> ()  [unwired: 1 out]
                      }
                    }
                  }
                  frame True {
                    n418 = local read "Large/Steel 1"() -> (w1831:dbl)
                    n419 = Decrement(x=w1831) -> (x-1=w1830:dbl)
                    n420 = local write "Large/Steel 1"(w1830) -> ()
                    n421 = xnode "Motors"() -> ("Motor"=w1815:T1)
                    n422 = xnode "Move a Fixed Distance"("Speed 1"=i8 75, "Distance 1"=360, "Motors"=w1815) -> ("NXT/EV3"=w1818:T3)  [unwired: 1 in]
                    n423 = xnode "Motors"() -> ("Motor"=w1819:T1)
                    n424 = xnode "Move a Fixed Distance"("Speed 1"=i8 -50, "Distance 1"=90, "Motors"=w1819, "NXT/EV3"=w1818) -> ("NXT/EV3"=w1829:T3)
                    n425 = xnode "Motors"() -> ("Motor"=w1825:T1)
                    n426 = xnode "Move a Fixed Distance"("Speed 1"=i8 -75, "Distance 1"=360, "Motors"=w1825, "NXT/EV3"=w1829) -> ("NXT/EV3"=w1828:T3)
                    n427 = xnode "Motors"() -> ("Motor"=w1822:T1)
                    n428 = xnode "Move a Fixed Distance"("Speed 1"=i8 50, "Distance 1"=90, "Motors"=w1822, "NXT/EV3"=w1828) -> ()  [unwired: 1 out]
                  }
                }
              }
              frame "Red Glass" {
                n429 = local read "Large/Steel 1"() -> (w1878:dbl)
                n430 = Greater?(x=w1878, y=0.0) -> (0:w1877:bool)
                n431 = case shown="False" w1877 {
                  frame False {
                    n432 = local read "Small/HDPE 1"() -> (w1881:dbl)
                    n433 = Greater?(x=w1881, y=0.0) -> (0:w1879:bool)
                    n434 = case shown="True" w1879 {
                      frame False {
                        (unwired) "donezo"
                      }
                      frame True {
                        n435 = xnode "Motors"() -> ("Motor"=w1882:T1)
                        n436 = local read "Small/HDPE 1"() -> (w1898:dbl)
                        n437 = xnode "Move a Fixed Distance"("Speed 1"=i8 75, "Distance 1"=360, "Motors"=w1882) -> ("NXT/EV3"=w1885:T3)  [unwired: 1 in]
                        n438 = Decrement(x=w1898) -> (x-1=w1897:dbl)
                        n439 = local write "Small/HDPE 1"(w1897) -> ()
                        n440 = xnode "Motors"() -> ("Motor"=w1886:T1)
                        n441 = xnode "Move a Fixed Distance"("Speed 1"=i8 -50, "Distance 1"=90, "Motors"=w1886, "NXT/EV3"=w1885) -> ("NXT/EV3"=w1896:T3)
                        n442 = xnode "Motors"() -> ("Motor"=w1892:T1)
                        n443 = xnode "Move a Fixed Distance"("Speed 1"=i8 -75, "Distance 1"=360, "Motors"=w1892, "NXT/EV3"=w1896) -> ("NXT/EV3"=w1895:T3)
                        n444 = xnode "Motors"() -> ("Motor"=w1889:T1)
                        n445 = xnode "Move a Fixed Distance"("Speed 1"=i8 50, "Distance 1"=90, "Motors"=w1889, "NXT/EV3"=w1895) -> ()  [unwired: 1 out]
                      }
                    }
                  }
                  frame True {
                    n446 = local read "Large/Steel 1"() -> (w1959:dbl)
                    n447 = xnode "Motors"() -> ("Motor"=w1943:T1)
                    n448 = Decrement(x=w1959) -> (x-1=w1958:dbl)
                    n449 = xnode "Move a Fixed Distance"("Speed 1"=i8 75, "Distance 1"=360, "Motors"=w1943) -> ("NXT/EV3"=w1946:T3)  [unwired: 1 in]
                    n450 = local write "Large/Steel 1"(w1958) -> ()
                    n451 = xnode "Motors"() -> ("Motor"=w1947:T1)
                    n452 = xnode "Move a Fixed Distance"("Speed 1"=i8 -50, "Distance 1"=90, "Motors"=w1947, "NXT/EV3"=w1946) -> ("NXT/EV3"=w1957:T3)
                    n453 = xnode "Motors"() -> ("Motor"=w1953:T1)
                    n454 = xnode "Move a Fixed Distance"("Speed 1"=i8 -75, "Distance 1"=360, "Motors"=w1953, "NXT/EV3"=w1957) -> ("NXT/EV3"=w1956:T3)
                    n455 = xnode "Motors"() -> ("Motor"=w1950:T1)
                    n456 = xnode "Move a Fixed Distance"("Speed 1"=i8 50, "Distance 1"=90, "Motors"=w1950, "NXT/EV3"=w1956) -> ()  [unwired: 1 out]
                  }
                }
              }
              frame "Blue Glass" {
                n457 = local read "Large/Steel 1"() -> (w2006:dbl)
                n458 = Greater?(x=w2006, y=0.0) -> (0:w2004:bool)
                n459 = case shown="True" w2004 {
                  frame False {
                    n460 = local read "Small/HDPE 1"() -> (w2008:dbl)
                    n461 = Greater?(x=w2008, y=0.0) -> (0:w2009:bool)
                    n462 = case shown="True" w2009 {
                      frame False {
                        (unwired) "Welcome to labview hell"
                      }
                      frame True {
                        n463 = local read "Small/HDPE 1"() -> (w2026:dbl)
                        n464 = xnode "Motors"() -> ("Motor"=w2010:T1)
                        n465 = xnode "Move a Fixed Distance"("Speed 1"=i8 75, "Distance 1"=360, "Motors"=w2010) -> ("NXT/EV3"=w2013:T3)  [unwired: 1 in]
                        n466 = Decrement(x=w2026) -> (x-1=w2025:dbl)
                        n467 = xnode "Motors"() -> ("Motor"=w2014:T1)
                        n468 = xnode "Move a Fixed Distance"("Speed 1"=i8 -50, "Distance 1"=90, "Motors"=w2014, "NXT/EV3"=w2013) -> ("NXT/EV3"=w2024:T3)
                        n469 = local write "Small/HDPE 1"(w2025) -> ()
                        n470 = xnode "Motors"() -> ("Motor"=w2020:T1)
                        n471 = xnode "Move a Fixed Distance"("Speed 1"=i8 -75, "Distance 1"=360, "Motors"=w2020, "NXT/EV3"=w2024) -> ("NXT/EV3"=w2023:T3)
                        n472 = xnode "Motors"() -> ("Motor"=w2017:T1)
                        n473 = xnode "Move a Fixed Distance"("Speed 1"=i8 50, "Distance 1"=90, "Motors"=w2017, "NXT/EV3"=w2023) -> ()  [unwired: 1 out]
                      }
                    }
                  }
                  frame True {
                    n474 = local read "Large/Steel 1"() -> (w2087:dbl)
                    n475 = xnode "Motors"() -> ("Motor"=w2071:T1)
                    n476 = xnode "Move a Fixed Distance"("Speed 1"=i8 75, "Distance 1"=360, "Motors"=w2071) -> ("NXT/EV3"=w2074:T3)  [unwired: 1 in]
                    n477 = Decrement(x=w2087) -> (x-1=w2086:dbl)
                    n478 = local write "Large/Steel 1"(w2086) -> ()
                    n479 = xnode "Motors"() -> ("Motor"=w2075:T1)
                    n480 = xnode "Move a Fixed Distance"("Speed 1"=i8 -50, "Distance 1"=90, "Motors"=w2075, "NXT/EV3"=w2074) -> ("NXT/EV3"=w2085:T3)
                    n481 = xnode "Motors"() -> ("Motor"=w2081:T1)
                    n482 = xnode "Move a Fixed Distance"("Speed 1"=i8 -75, "Distance 1"=360, "Motors"=w2081, "NXT/EV3"=w2085) -> ("NXT/EV3"=w2084:T3)
                    n483 = xnode "Motors"() -> ("Motor"=w2078:T1)
                    n484 = xnode "Move a Fixed Distance"("Speed 1"=i8 50, "Distance 1"=90, "Motors"=w2078, "NXT/EV3"=w2084) -> ()  [unwired: 1 out]
                  }
                }
              }
              frame "Steel/HDPE" {
                n485 = local read "Large/Steel 1"() -> (w2134:dbl)
                n486 = Greater?(x=w2134, y=0.0) -> (0:w2133:bool)
                n487 = case shown="False" w2133 {
                  frame False {
                    n488 = local read "Small/HDPE 1"() -> (w2137:dbl)
                    n489 = Greater?(x=w2137, y=0.0) -> (0:w2136:bool)
                    n490 = case shown="True" w2136 {
                      frame False {
                        (unwired) "why are you even here"
                      }
                      frame True {
                        n491 = local read "Small/HDPE 1"() -> (w2154:dbl)
                        n492 = xnode "Motors"() -> ("Motor"=w2138:T1)
                        n493 = Decrement(x=w2154) -> (x-1=w2153:dbl)
                        n494 = xnode "Move a Fixed Distance"("Speed 1"=i8 75, "Distance 1"=360, "Motors"=w2138) -> ("NXT/EV3"=w2141:T3)  [unwired: 1 in]
                        n495 = local write "Small/HDPE 1"(w2153) -> ()
                        n496 = xnode "Motors"() -> ("Motor"=w2142:T1)
                        n497 = xnode "Move a Fixed Distance"("Speed 1"=i8 -50, "Distance 1"=90, "Motors"=w2142, "NXT/EV3"=w2141) -> ("NXT/EV3"=w2152:T3)
                        n498 = xnode "Motors"() -> ("Motor"=w2148:T1)
                        n499 = xnode "Move a Fixed Distance"("Speed 1"=i8 -75, "Distance 1"=360, "Motors"=w2148, "NXT/EV3"=w2152) -> ("NXT/EV3"=w2151:T3)
                        n500 = xnode "Motors"() -> ("Motor"=w2145:T1)
                        n501 = xnode "Move a Fixed Distance"("Speed 1"=i8 50, "Distance 1"=90, "Motors"=w2145, "NXT/EV3"=w2151) -> ()  [unwired: 1 out]
                      }
                    }
                  }
                  frame True {
                    n502 = local read "Large/Steel 1"() -> (w2215:dbl)
                    n503 = Decrement(x=w2215) -> (x-1=w2214:dbl)
                    n504 = xnode "Motors"() -> ("Motor"=w2199:T1)
                    n505 = xnode "Move a Fixed Distance"("Speed 1"=i8 75, "Distance 1"=360, "Motors"=w2199) -> ("NXT/EV3"=w2202:T3)  [unwired: 1 in]
                    n506 = local write "Large/Steel 1"(w2214) -> ()
                    n507 = xnode "Motors"() -> ("Motor"=w2203:T1)
                    n508 = xnode "Move a Fixed Distance"("Speed 1"=i8 -50, "Distance 1"=90, "Motors"=w2203, "NXT/EV3"=w2202) -> ("NXT/EV3"=w2213:T3)
                    n509 = xnode "Motors"() -> ("Motor"=w2209:T1)
                    n510 = xnode "Move a Fixed Distance"("Speed 1"=i8 -75, "Distance 1"=360, "Motors"=w2209, "NXT/EV3"=w2213) -> ("NXT/EV3"=w2212:T3)
                    n511 = xnode "Motors"() -> ("Motor"=w2206:T1)
                    n512 = xnode "Move a Fixed Distance"("Speed 1"=i8 50, "Distance 1"=90, "Motors"=w2206, "NXT/EV3"=w2212) -> ()  [unwired: 1 out]
                  }
                }
              }
            }
          }
        }
      }
    }
  }
